vi "Global Elapsed time.vi"() -> ()   [LabVIEW 2017]
panel:
  in  "Elapsed Time":dbl
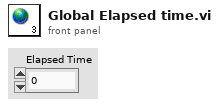
[diagram p1: front panel]
diagram:
